vi "initializeValveSerial-v01.vi"(8 "error in":errorcluster, 11 "Valve COM":refnum<visa-resource-name>="COM1") -> (0 "error out":errorcluster, 2 "ValveSetTo":u16, 3 "VISA resource name out":refnum<visa-resource-name>)   [LabVIEW 2015]
uses:
  <vilib>/Instr/_visa.llb/VISA Configure Serial Port (Serial Instr).vi
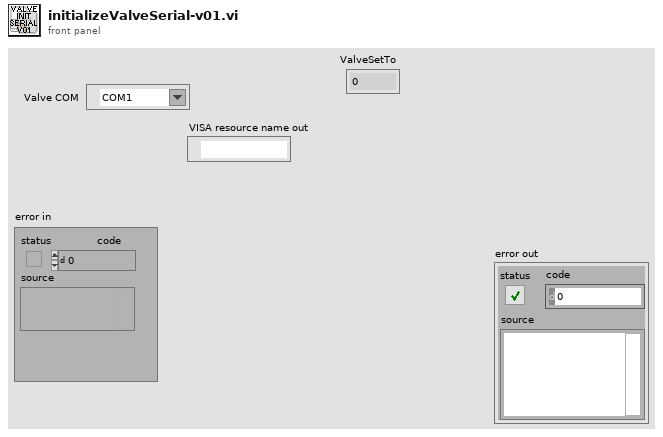
[diagram p1: front panel]
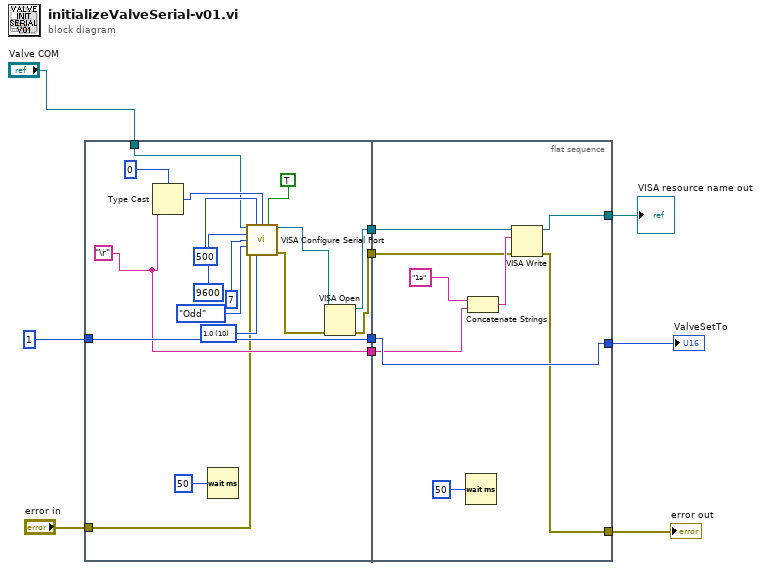
[diagram p0: block diagram]
diagram:
  n1 = flat-sequence {
    tunnel: "Valve COM" -> [w12]
    tunnel: u16 1 -> [w26]
    tunnel: [w26] -> w10
    tunnel: "error in" -> [w11]
    tunnel: [w15] -> w5
    tunnel: [w14] -> w3
    tunnel: [w13] -> w1
    tunnel: w10 -> [w36]
    tunnel: [w36] -> w9
    tunnel: w5 -> [w33]
    tunnel: [w32] -> w4
    tunnel: w3 -> [w31]
    tunnel: [w30] -> w2
    tunnel: w1 -> [w29]
    frame #0 {
      w13 = "\r"
      w20 = u16 10 items=["1.0"=10, "1.5"=15, "2.0"=20] ("stop bits (10: 1 bit)")
      n2 = Type Cast(type=u8 0, x=w13) -> (*(type *) &x=w25:u8)
      n3 = Wait (ms)(milliseconds to wait=u32 50) -> ()  [unwired: 1 out]
      n4 = call-poly "VISA Configure Serial Port"("VISA resource name"=w12, "timeout (10sec)"=u32 500, "termination char\n(0xA = '\\n' = LF)"=w25, "Enable Termination\nChar (T)"=TRUE ("Enable Termination\nChar (T)"), "baud rate (9600)"=u32 9600, "data bits (8)"=u16 7, "parity (0:none)"=enum16{"None", "Odd", "Even", "Mark", "Space"}."Odd", "error in (no error)"=w11, "stop bits (10: 1 bit)"=w20) -> ("VISA resource name out"=w16:refnum<visa-resource-name>, "error out"=w17:errorcluster)  [unwired: 5 in]
      n5 = VISA Open(error in (no error)=w17, VISA resource name=w16) -> (VISA resource name=w15:refnum<visa-resource-name>, error out=w14:errorcluster)  [unwired: 3 in]
    }
    frame #1 {
      n6 = Wait (ms)(milliseconds to wait=u32 50) -> ()  [unwired: 1 out]
      n7 = Concatenate Strings("1a" ("write buffer"), w29) -> (w35:string)
      n8 = VISA Write(VISA resource name=w33, write buffer=w35, error in (no error)=w31) -> (VISA resource name out=w32:refnum<visa-resource-name>, error out=w30:errorcluster)  [unwired: 1 out]
    }
  }
  "ValveSetTo" <- w9
  "error out" <- w2
  "VISA resource name out" <- w4
